vi "yaq_labview_error_handler.vi"(8 "error in (no error)":errorcluster) -> (0 "error out":errorcluster)   [LabVIEW 2022 SP3]
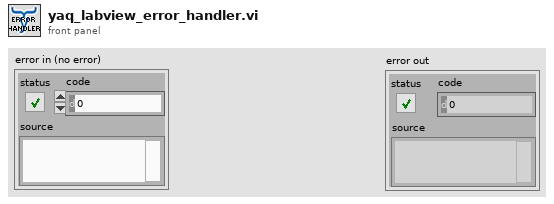
[diagram p1: front panel]
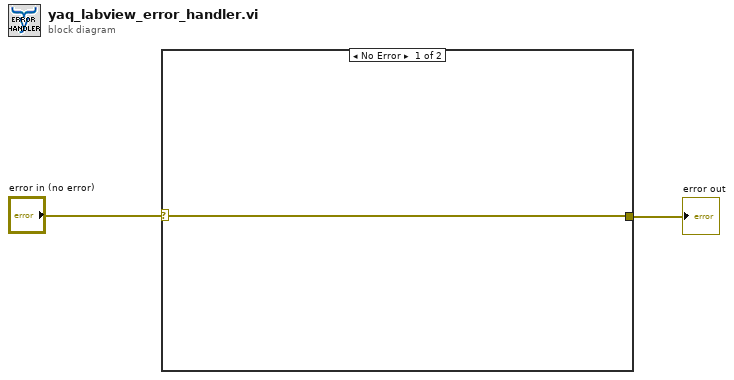
[diagram p0: block diagram]
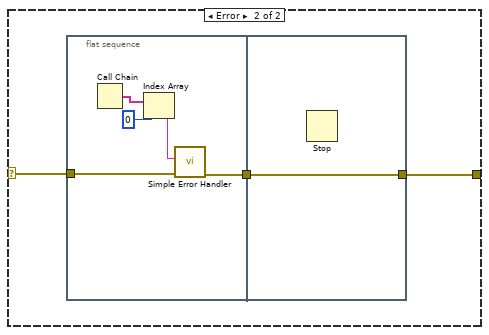
[diagram p2: hidden frame]
diagram:
  n1 = case shown="No Error" "error in (no error)" {
    selector: "error in (no error)" -> [w3 w6]
    tunnel: [w3 w5] -> w1
    frame No Error {
    }
    frame Error {
      n2 = flat-sequence {
        tunnel: w6 -> [w11]
        tunnel: [w10] -> w4
        tunnel: [w12] -> w5
        tunnel: w4 -> [w12]
        frame #0 {
          n3 = Call Chain() -> (call chain=w9:string[])
          n4 = Index Array(array=w9, index=0) -> (element=w7:string)
          n5 = call <vilib>:"Simple Error Handler.vi"("error source (\" \")"=w7, "error in (no error)"=w11) -> ("error out"=w10:errorcluster)  [unwired: 3 in, 4 out]
        }
        frame #1 {
          n6 = Stop() -> ()  [unwired: 1 in]
        }
      }
    }
  }
  "error out" <- w1
